vi "getModbusSubnetA.vi"(11 "Model in":refnum<class "Model.lvclass">) -> (2 "Modbus":refnum<class "IModbus.lvclass">, 3 "Model out":refnum<class "Model.lvclass">)   [LabVIEW 2016]
uses:
  Model.lvclass
  Common_RT_Modbus/IModbus/IModbus.lvclass
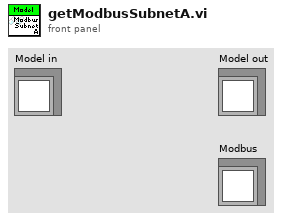
[diagram p1: front panel]
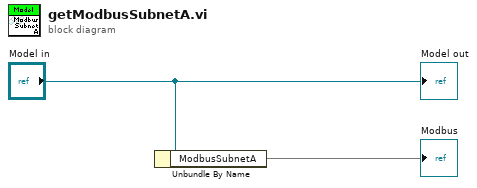
[diagram p0: block diagram]
diagram:
  n1 = Unbundle By Name("Model in") -> ("ModbusSubnetA"=→"Modbus")
  "Model out" <- "Model in"
